vi "waveform simulator.vi"(1 "Amplitude":dbl, 2 "Frequency":dbl) -> (0 "Waveform Graph":dynamicdata(graph))   [LabVIEW 2015]
uses:
  <vilib>/Utility/file.llb/Write Delimited Spreadsheet (DBL).vi
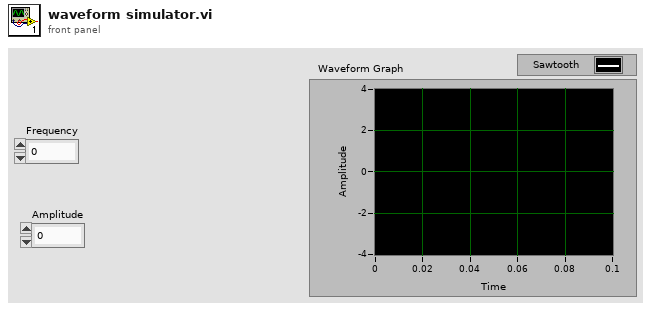
[diagram p1: front panel]
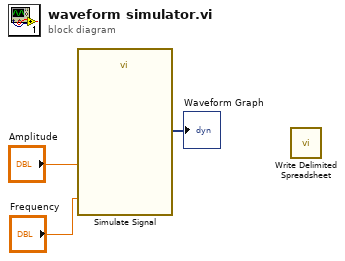
[diagram p0: block diagram]
diagram:
  n1 = call "Simulate Signal"("Frequency"="Frequency", "Amplitude"="Amplitude") -> ("Sawtooth"=→"Waveform Graph":dynamicdata)  [unwired: 12 in, 1 out]
  n2 = call-poly <vilib>:"Write Delimited Spreadsheet.vi"() -> ()  [unwired: 14 in, 2 out]
